vi "Set View FP State.vi"(0 "GUI Container in":refnum<class "GUI Container.lvclass">, 5 "View":string, 7 "View Hierarchy Level":i32, 9 "Front Panel Window:State":T1(ring), 11 "error in (no error)":errorcluster) -> (4 "GUI Container out":refnum<class "GUI Container.lvclass">, 15 "error out":errorcluster)   [LabVIEW 2023, in "GUI Views.lvlib" / "GUI Container.lvclass"]
doc: "Sets the state of the Front Panel of a specified Actor Core VI of the the specified View class hierarchy. The Front Panel is specified by: \n\n<b> View </b> String theat contains the name of the View\n\n<b> View Hierarchy Level</b> the level on the subclassing hierarchy of the GUI View actor, it is used to choose the Actor Core Front Panel among all the exisiting sublcasses of the GUI VIew Actor present in the View specified above"
uses:
  GUI Container.lvclass
  GUI Container.lvclass/GUI Container.ctl
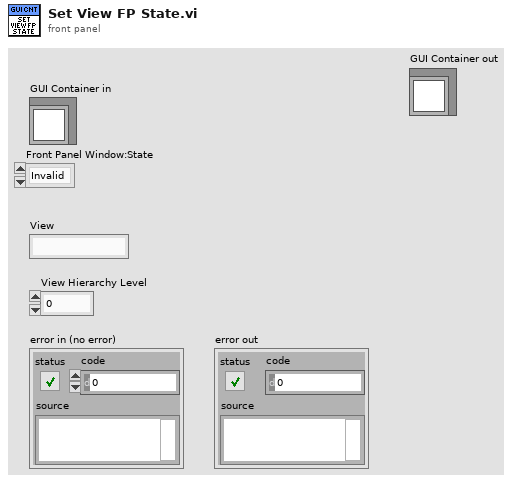
[diagram p1: front panel]
types:
  T1 = enum32{"Invalid", "Standard", "Closed", "Hidden", "Minimized", "Maximized"}
  T2 = typedef "GUI Views.lvlib/GUI Container.lvclass/View Status.ctl" = cluster{"View Details":T3, "Front Panel Statuses":T4[]}
  T3 = typedef "GUI Views.lvlib/GUI Container.lvclass/View Details.ctl" = cluster{"Enqueuer":refnum<class "Message Enqueuer.lvclass">, "VI References":refnum<vi>[], "FP References":refnum<vi>[]}
  T4 = typedef "GUI Views.lvlib/GUI Container.lvclass/FP Status.ctl" = cluster{"FP Open":bool, "Inserted in Subpanel":bool, "Subpanel":string}
  T5 = typedef "GUI Views.lvlib/GUI Container.lvclass/VI References.ctl" = cluster{"FP Ref":refnum<vi>, "VI Ref":refnum<vi>}
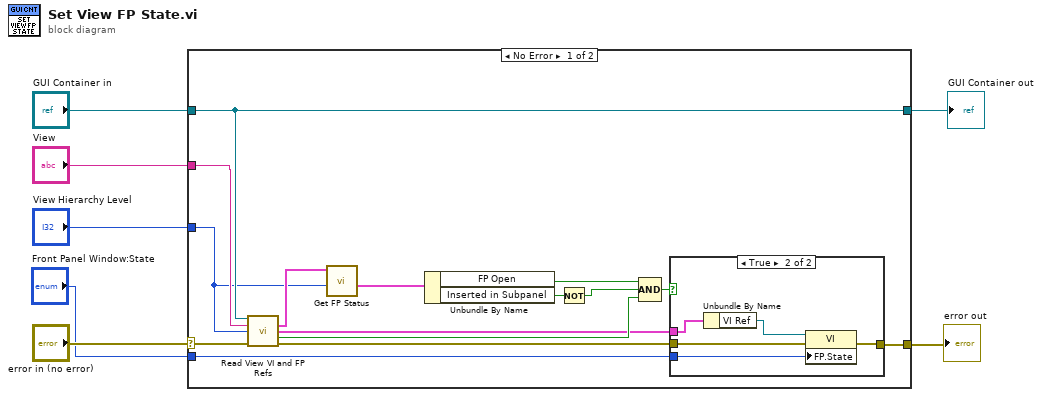
[diagram p0: block diagram]
diagram:
  n1 = case shown="No Error" "error in (no error)" {
    selector: "error in (no error)" -> [w20 w29]
    tunnel: [w22 w29] -> w7
    tunnel: "GUI Container in" -> [w18 w30]
    tunnel: "View Hierarchy Level" -> [w9 _]
    tunnel: "View" -> [w17 _]
    tunnel: [w18 w30] -> w2
    tunnel: "Front Panel Window:State" -> [w21 _]
    frame No Error {
      n2 = call "Read View VI and FP Refs.vi"("GUI Container Actor in"=w18, "View"=w17, "View Hierarchy Level"=w9, "error in (no error)"=w20) -> ("View Status"=w11:T2, "VI References"=w8:T5, "View Found"=w15:bool, "error out"=w19:errorcluster)  [unwired: 7 in, 1 out]
      n3 = call "Get FP Status.vi"("View Hierarchy Level"=w9, "View Status in"=w11) -> ("FP Status"=w10:T4)  [unwired: 8 in, 1 out]
      n4 = Unbundle By Name(w10) -> ("FP Open"=w16:bool, "Inserted in Subpanel"=w13:bool)
      n5 = Not(x=w13) -> (.not. x?=w12:bool)
      n6 = Compound Arithmetic op=AND(w16, w12, w15) -> (w14:bool)
      n7 = case shown="True" w14 {
        tunnel: [w23 w28] -> w22
        tunnel: w21 -> [_ w27]
        tunnel: w19 -> [w23 w26]
        tunnel: w8 -> [_ w25]
        frame False {
        }
        frame True {
          n8 = Unbundle By Name(w25) -> ("VI Ref"=w24:refnum<vi>)
          n9 = property class="VI"(reference=w24, error in=w26, "FP.State"=w27) -> (error out=w28:errorcluster)  [unwired: 1 out]
        }
      }
    }
    frame Error {
    }
  }
  "error out" <- w7
  "GUI Container out" <- w2
